vi "Sequence Inputs.vi"(6 "Time In":dbl, 8 "error in":errorcluster, 10 "Actuation Array in":bool[](array[boolean]), 11 "Sequence":T1(array[cluster])) -> (0 "error out":errorcluster, 2 "Actuation Array out":bool[](array[boolean]))   [LabVIEW 2024]
panel:
  in  "Time Buffer":dbl=1.0 format="%#_13g"
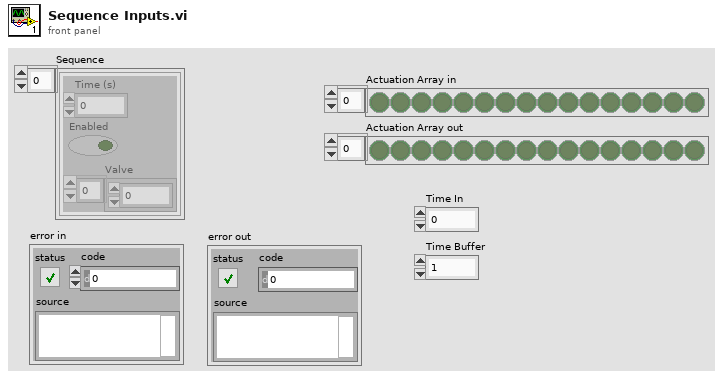
[diagram p1: front panel]
types:
  T1 = cluster{"Time (s)":dbl, "Enabled":bool, "Valve":u16[]}[]
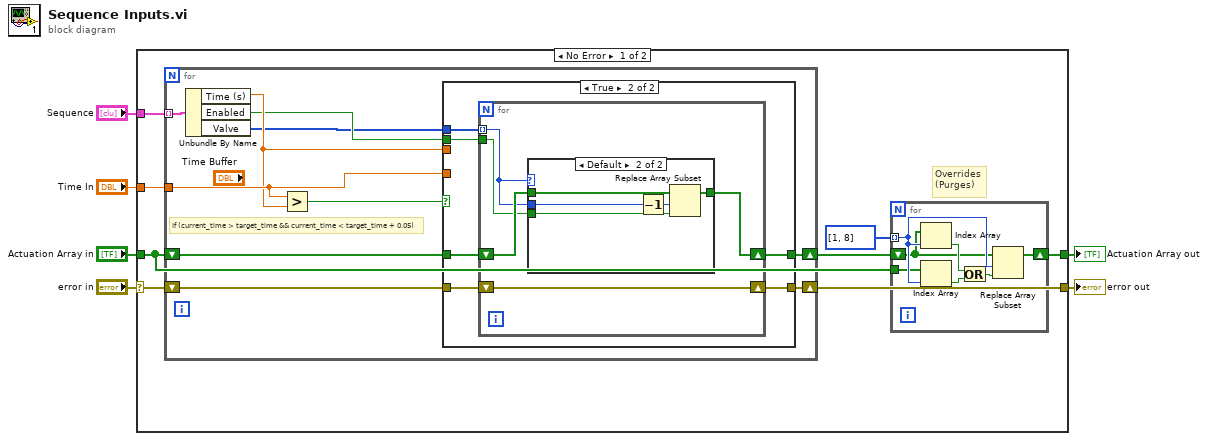
[diagram p0: block diagram]
diagram:
  n1 = case shown="No Error" "error in" {
    selector: "error in" -> [w12 w52]
    tunnel: [w11 w52] -> w5
    tunnel: "Time In" -> [w14 _]
    tunnel: "Actuation Array in" -> [w7 w51]
    tunnel: [w9 w51] -> w3
    tunnel: "Sequence" -> [w13 _]
    frame No Error {
      # "Overrides\n(Purges)"
      n2 = for {
        tunnel: w14 -> [w30]
        tunnel: w13 -> [w31] mode=indexing
        shift-right: [w24] -> w11
        shift-left: w12 -> [w25]
        shift-right: [w23] -> w10
        shift-left: w7 -> [w26]
        # "If (current_time > target_time && current_time < target_time + 0.05)"
        n3 = Unbundle By Name(w31) -> ("Time (s)"=w29:dbl, "Enabled"=w28:bool, "Valve"=w27:u16[])
        n4 = Greater?(x=w30, y=w29) -> (0:w22:bool)
        n5 = case shown="True" w22 {
          tunnel: w30 -> [_ _]
          tunnel: w29 -> [_ _]
          tunnel: w28 -> [_ w34]
          tunnel: w27 -> [_ w35]
          tunnel: w26 -> [w32 w37]
          tunnel: w25 -> [w33 w39]
          tunnel: [w33 w38] -> w24
          tunnel: [w32 w36] -> w23
          frame False {
          }
          frame True {
            n6 = for {
              shift-right: [w44] -> w38
              shift-left: w39 -> [w44]
              shift-right: [w43] -> w36
              shift-left: w37 -> [w42]
              tunnel: w35 -> [w40] mode=indexing
              tunnel: w34 -> [w41]
              n7 = case shown="Default" w40 {
                tunnel: [w45 w50] -> w43
                tunnel: w42 -> [w45 w49]
                tunnel: w41 -> [_ w48]
                tunnel: w40 -> [_ w46]
                frame 0 {
                }
                frame Default {
                  n8 = Decrement(x=w46) -> (x-1=w47:u16)
                  n9 = Replace Array Subset(array=w49, new element=w48, index=w47) -> (w50:bool[])
                }
              }
            }
          }
        }
      }
      n10 = for {
        shift-right: [w21] -> w9
        shift-left: w10 -> [w15]
        tunnel: i32[] [1, 8] -> [w17] mode=indexing
        tunnel: w7 -> [w16]
        n11 = Index Array(array=w15, index=w17) -> (element=w18:bool)
        n12 = Index Array(array=w16, index=w17) -> (element=w19:bool)
        n13 = Or(x=w18, y=w19) -> (x .or. y?=w20:bool)
        n14 = Replace Array Subset(array=w15, new element=w20, index=w17) -> (w21:bool[])
      }
    }
    frame Error {
    }
  }
  "error out" <- w5
  "Actuation Array out" <- w3
